vi "DS3231_Get_PC_Date_Time.vi"() -> (0 "DS3231_Friendly_Array":u8[](array[numeric]), 3 "PC_Date_Time":T1)   [LabVIEW 2022 SP3]
uses:
  DS3231_Date_Time.ctl
  <vilib>/MakerHub/Toolbox/LMH-Toolbox.lvlib
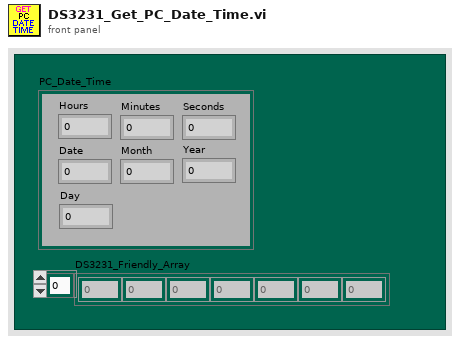
[diagram p1: front panel]
types:
  T1 = typedef "DS3231_Date_Time.ctl" = cluster{"Seconds":u8, "Minutes":u8, "Hours":u8, "Day":u8, "Date":u8, "Month":u8, "Year":u8}
  T2 = typedef "LVDateTimeRec.ctl" = cluster{"fractional second":dbl, "second":i32, "minute":i32, "hour":i32, "day of month":i32, "month":i32, "year":i32, "day of week":i32, "day of year":i32, "DST":i32}
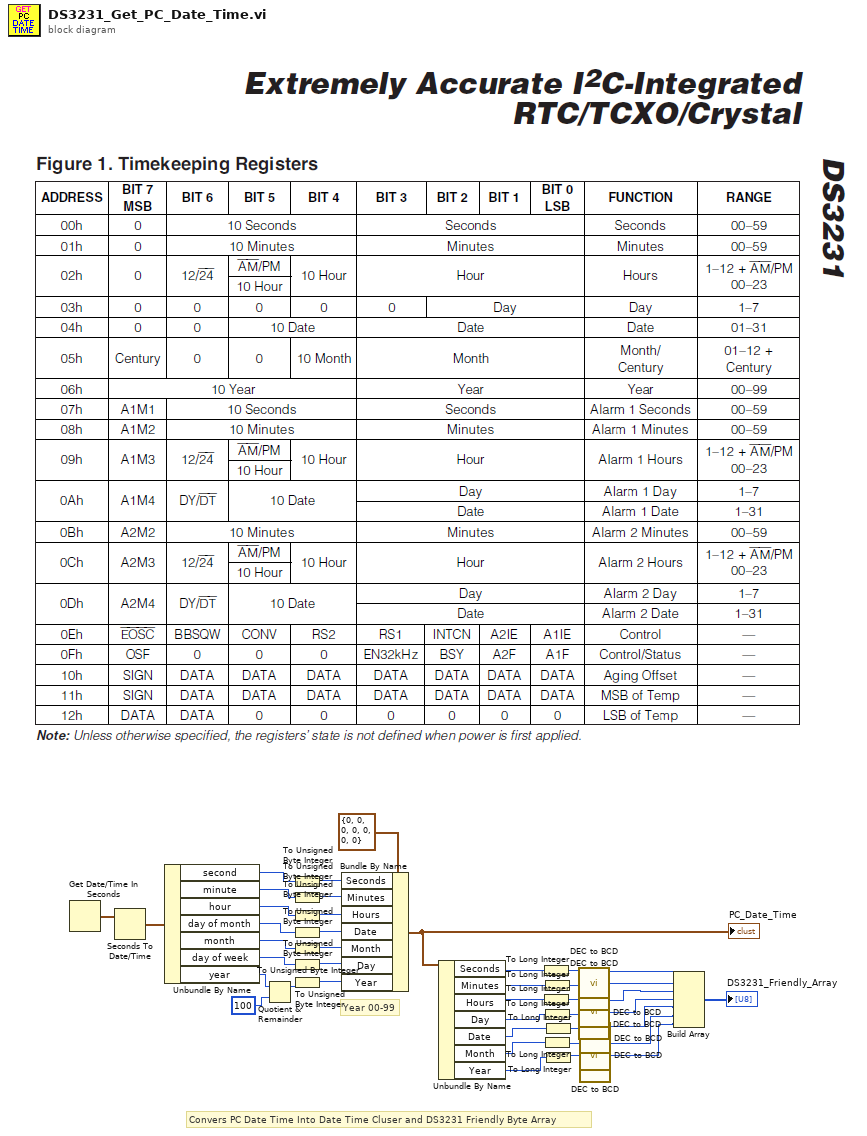
[diagram p0: block diagram]
diagram:
  # "Convers PC Date Time Into Date Time Cluser and DS3231 Friendly Byte Array"
  # "Year 00-99"
  n1 = Get Date/Time In Seconds() -> (seconds since 1Jan1904=w31:timestamp)
  n2 = Seconds To Date/Time(time stamp (now)=w31) -> (date time rec=w32:T2)  [unwired: 1 in]
  n3 = Unbundle By Name(w32) -> ("second"=w33:i32, "minute"=w34:i32, "hour"=w35:i32, "day of month"=w36:i32, "month"=w37:i32, "day of week"=w38:i32, "year"=w39:i32)
  n4 = Quotient & Remainder(x=w39, y=100) -> (x-y*floor(x/y)=w41:i32)  [unwired: 1 out]
  n5 = To Unsigned Byte Integer(number=w33) -> (unsigned 8bit integer=w27:u8)
  n6 = To Unsigned Byte Integer(number=w34) -> (unsigned 8bit integer=w25:u8)
  n7 = To Unsigned Byte Integer(number=w35) -> (unsigned 8bit integer=w17:u8)
  n8 = To Unsigned Byte Integer(number=w36) -> (unsigned 8bit integer=w16:u8)
  n9 = To Unsigned Byte Integer(number=w37) -> (unsigned 8bit integer=w15:u8)
  n10 = To Unsigned Byte Integer(number=w38) -> (unsigned 8bit integer=w14:u8)
  n11 = To Unsigned Byte Integer(number=w41) -> (unsigned 8bit integer=w13:u8)
  n12 = Bundle By Name(cluster=T1 {"Seconds"=0, "Minutes"=0, "Hours"=0, "Day"=0, "Date"=0, "Month"=0, "Year"=0} ("PC_Date_Time"), "Seconds"=w27, "Minutes"=w25, "Hours"=w17, "Date"=w16, "Month"=w15, "Day"=w14, "Year"=w13) -> (w8:T1)
  "PC_Date_Time" <- w8
  n13 = Unbundle By Name(w8) -> ("Seconds"=w7:u8, "Minutes"=w6:u8, "Hours"=w5:u8, "Day"=w4:u8, "Date"=w3:u8, "Month"=w2:u8, "Year"=w1:u8)
  n14 = To Long Integer(number=w7) -> (32bit integer=w28:i32)
  n15 = To Long Integer(number=w5) -> (32bit integer=w24:i32)
  n16 = To Long Integer(number=w6) -> (32bit integer=w26:i32)
  n17 = To Long Integer(number=w4) -> (32bit integer=w23:i32)
  n18 = To Long Integer(number=w2) -> (32bit integer=w11:i32)
  n19 = To Long Integer(number=w3) -> (32bit integer=w12:i32)
  n20 = To Long Integer(number=w1) -> (32bit integer=w10:i32)
  n21 = call <vilib>:"DEC to BCD.vi"("DEC"=w28) -> ("BCD"=w30:u8)  [unwired: 10 in]
  n22 = call <vilib>:"DEC to BCD.vi"("DEC"=w26) -> ("BCD"=w29:u8)  [unwired: 10 in]
  n23 = call <vilib>:"DEC to BCD.vi"("DEC"=w24) -> ("BCD"=w22:u8)  [unwired: 10 in]
  n24 = call <vilib>:"DEC to BCD.vi"("DEC"=w23) -> ("BCD"=w21:u8)  [unwired: 10 in]
  n25 = call <vilib>:"DEC to BCD.vi"("DEC"=w12) -> ("BCD"=w20:u8)  [unwired: 10 in]
  n26 = call <vilib>:"DEC to BCD.vi"("DEC"=w11) -> ("BCD"=w19:u8)  [unwired: 10 in]
  n27 = call <vilib>:"DEC to BCD.vi"("DEC"=w10) -> ("BCD"=w18:u8)  [unwired: 10 in]
  n28 = Build Array(w30, w29, w22, w21, w20, w19, w18) -> (→"DS3231_Friendly_Array":u8[])
